vi "test_template_serializedandclusterconstructorsconstructors_appliedcorrectly.vi"   [LabVIEW 2020]
doc: "Checks whether the PE is able to load, and whether the serialize and deserialize functions can successfully apply and return a configuration."
uses:
  PE/Configuration.ctl
  PE/ADAS PE Template.lvclass/ADAS PE Template.ctl
  PE/Read Configuration.vi
  PE/Write Configuration Parameter.vi
  PE/Get Configuration Version.vi
  PE/Write Serialized Configuration Parameter.vi
  PE/ADAS PE Template.lvclass
  C:/Program Files/National Instruments/LabVIEW 2020/vi.lib/FlexLogger/SDK/PluginSDK.lvlibp/PEFClasses/SDK/Processing Element/Processing Element.lvclass
  <vilib>/ADAS Record/Utilities/Config/Data Converter/Data Container and Version to JSON.vi
  <vilib>/FlexLogger/SDK/PluginSDK.lvlibp/PEFClasses/SDK/Processing Element/Read Parameters Property.vi
  <vilib>/FlexLogger/SDK/PluginSDK.lvlibp/PEFClasses/SDK/Parameters/Set Parameter.vi
  <vilib>/FlexLogger/SDK/PluginSDK.lvlibp/PEFClasses/SDK/Parameters/SetParameter(String).vi
  <vilib>/FlexLogger/SDK/PluginSDK.lvlibp/PEFClasses/SDK/Processing Element/Write Parameters Property.vi
  <vilib>/FlexLogger/SDK/PluginSDK.lvlibp/PEFClasses/SDK/Parameters/Parameters.lvclass
  <vilib>/addons/_JKI Toolkits/Caraya/classes/Test/Test.lvclass
  <vilib>/addons/_JKI Toolkits/Caraya/classes/Assert/Assert.lvclass
types:
  T1 = typedef "ADAS PE Template.lvlib/ADAS PE Template.lvclass/Configuration.ctl" = cluster{"Parameter1":string}
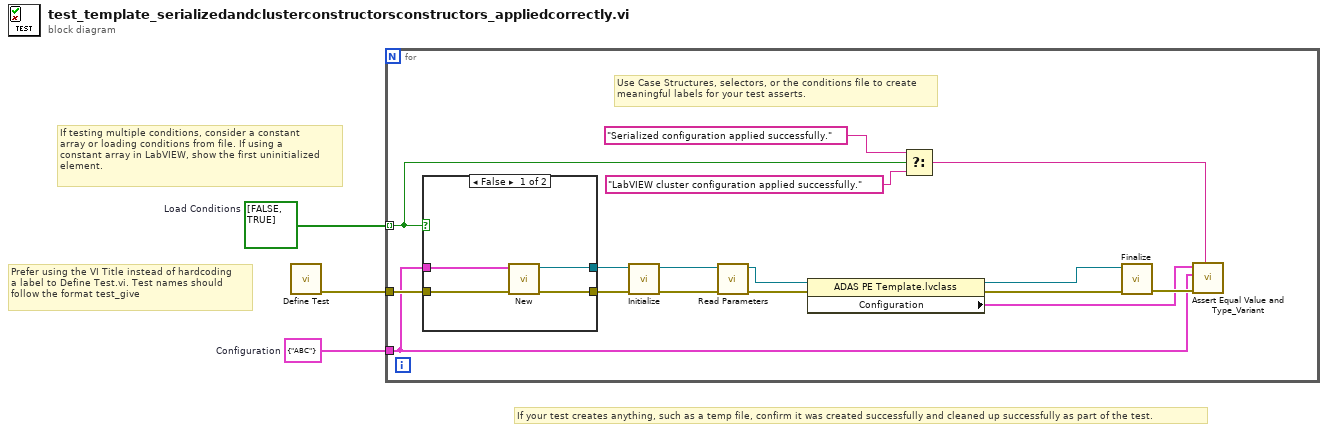
[diagram p0: block diagram]
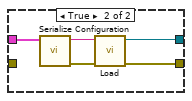
[diagram p2: hidden frame]
diagram:
  w1 = bool[] [FALSE, TRUE]  # Load Conditions
  w3 = T1 {"Parameter1"="ABC"}  # Configuration
  # "If your test creates anything, such as a temp file, confirm it was created successfully and cleaned up successfully as part of the test."
  # "Prefer using the VI Title instead of hardcoding\na label to Define Test.vi. Test names should\nfollow the format test_give"
  # "If testing multiple conditions, consider a constant\narray or loading conditions from file. If using a\nconstant array in LabVIEW, show the first uninitialized\nelement."
  n1 = call <vilib>:"Define Test.vi"() -> ("error out"=w2:errorcluster)  [unwired: 11 in]
  n2 = for {
    tunnel: w3 -> [w8]
    tunnel: w2 -> [w11]
    tunnel: w1 -> [w7] mode=indexing
    # "Use Case Structures, selectors, or the conditions file to create\nmeaningful labels for your test asserts."
    n3 = case shown="False" w7 {
      tunnel: [w23 w28] -> w18
      tunnel: [w22 w27] -> w17
      tunnel: w8 -> [w21 w25]
      tunnel: w11 -> [w20 _]
      frame False {
        n4 = call "New.vi"("error in (no error)"=w20, "Configuration"=w21) -> ("error out"=w23:errorcluster, "ADAS PE Template out"=w22:refnum<class "ADAS PE Template.lvclass">)  [unwired: 8 in]
      }
      frame True {
        n5 = call "Serialize Configuration.vi"("Configuration"=w25) -> ("error out"=w26:errorcluster, "Serialized Configuration"=w24:string)  [unwired: 9 in]
        n6 = call "Load.vi"("error in (no error)"=w26, "Serialized Configuration"=w24) -> ("error out"=w28:errorcluster, "ADAS PE Template out"=w27:refnum<class "ADAS PE Template.lvclass">)  [unwired: 8 in]
      }
    }
    n7 = call-dynamic "Initialize.vi"("error in (no error)"=w18, "ADAS PE Template in"=w17) -> ("error out"=w19:errorcluster, "ADAS PE Template out"=w15:refnum<class "ADAS PE Template.lvclass">)  [unwired: 8 in]
    n8 = call-dynamic "Read Parameters.vi"("error in (no error)"=w19, "ADAS PE Template in"=w15) -> ("error out"=w16:errorcluster, "ADAS PE Template out"=w13:refnum<class "ADAS PE Template.lvclass">)  [unwired: 7 in, 1 out]
    n9 = property class="ADAS PE Template.lvclass"(reference=w13, error in=w16) -> (reference out=w12:refnum<class "ADAS PE Template.lvclass">, error out=w14:errorcluster, "Configuration"=w9:T1)
    n10 = Select(t="Serialized configuration applied successfully.", s=w7, f="LabVIEW cluster configuration applied successfully.") -> (s? t:f=w4:string)
    n11 = call-dynamic "Finalize.vi"("error in (no error)"=w14, "ADAS PE Template in"=w12) -> ("error out"=w10:errorcluster)  [unwired: 8 in, 1 out]
    n12 = call <vilib>:"Assert Equal Value and Type_Variant.vi"("Label"=w4, "error in (no error)"=w10, "Y"=w8, "X"=w9) -> ()  [unwired: 7 in, 1 out]
  }
